vi "服务器更改对话框.vi"(11 "服务器信息":T1={"host"="27.154.58.30", "port"=8020, "user"="std", "password"="std23506", "远端地址"="/微站/四代/一体化微型水质监测站.exe"}) -> (2 "服务器信息 2":T1, 3 "check?":bool)   [LabVIEW 2016, in "数据传输系统-02.lvlib" / "update.lvlib"]
uses:
  update.lvlib
panel:
  in  "取消":bool
  in  "确认":bool
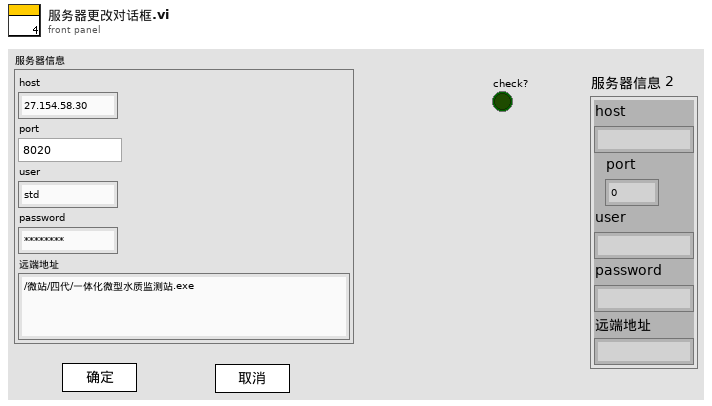
[diagram p1: front panel]
types:
  T1 = cluster{"host":string, "port":u16, "user":string, "password":string, "远端地址":string}
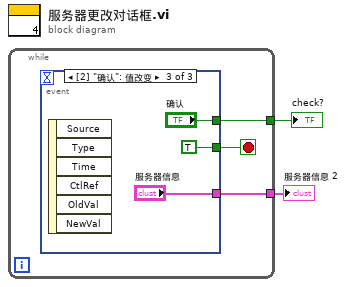
[diagram p0: block diagram]
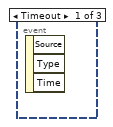
[diagram p2: hidden frame]
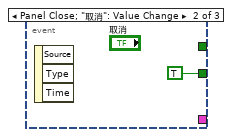
[diagram p3: hidden frame]
diagram:
  n1 = while {
    tunnel: [w4] -> w2
    tunnel: [w3] -> w1
    stop <- w5 stop-if-true
    n2 = event shown="[2] \"确认\": 值改变" {
      selector: _ -> [_ _ _]
      dyn-events: _ -> [_ _ _]
      timeout: _ -> [_ _ _]
      tunnel: [_ TRUE TRUE] -> w5
      tunnel: [_ _ "确认"] -> w4
      tunnel: [_ _ "服务器信息"] -> w3
      event Timeout {
        n3 = event-data() -> ()  [unwired: 1 in, 3 out]
      }
      event Panel Close; "取消": Value Change {
        n4 = event-data() -> ()  [unwired: 1 in, 3 out]
      }
      event "确认": Value Change {
        n5 = event-data() -> ()  [unwired: 1 in, 6 out]
      }
    }
  }
  "check?" <- w2
  "服务器信息 2" <- w1
